vi "Test NI DAQ API.vi"() -> ()   [LabVIEW 2020]
doc: "NI DAQ API Tester."
uses:
  NI DAQ.lvlib
  <vilib>/Utility/error.llb/DialogType.ctl
  <resource>/objmgr/daqmx.rc
  Support/Task list.ctl
  Support/Continuous aquisition params.ctl
  <vilib>/Utility/miscctls.llb/LVRowAndColumnTypeDef.ctl
  AI config parameters--cluster.ctl
panel:
  in  "Task list":T1 caption="Task"
  in  "Channels available":i32(listbox)
  out "Waveform Chart":dbl[](graph)
  out "Digital data":bool[](array[boolean])
  out "Analog data":dbl[](array[numeric])
  in  "Stop continuous acquisition":bool
  in  "N samples":i32
  in  "Acquisition type":enum16{"Single", "Multiple"}(ring)=enum."Multiple"
  in  "Start continous acquisition":bool
  out "DevSerialNum":u32
  out "Connection valid?":bool
  in  "Validate connection":bool
  in  "Sleep HL":bool
  in  "Task list":T1=enum."DO task" caption="Task"
  in  "Timeout":i32=100
  in  "Wake up HL":bool
  in  "Task list 2":T1 caption="Task to get"
  out "DAQmx Task":refnum<k21>
  in  "Get task ref":bool
  in  "Tab Control":enum32{"DO", "DI", "AI", "AO", "CI"}(tab)
  in  "Write DO":bool
  in  "Samples":enum16{"Single", "Multiple"}(ring)
  in  "Data":bool[](array[boolean])
  in  "Create DO channel":bool
  in  "Create DI channel":bool
  in  "Samples 2":enum16{"Single", "Multiple"}(ring) caption="Samples"
  in  "Read DI":bool
  out "Data read":bool[](array[boolean])
  in  "Create AI channel":bool
  in  "Config params":T2={"Terminal configuration"=-1, "min value"=-5.0, "max value"=5.0} {"max value" format="%0.2f"; "min value" format="%0.2f"; "Terminal configuration" items=["Default"=-1, "RSE"=10083, "NRSE"=10078, "Differential"=10106, "Pseudodifferential"=12529]}
  in  "Read AI":bool
  in  "Samples 3":enum16{"Single", "Multiple"}(ring) caption="Samples"
  out "AI Data":dbl[](array[numeric])
  in  "Create AO channel":bool
  in  "Config params 2":T2={"Terminal configuration"=-1, "min value"=-5.0, "max value"=5.0} caption="Config params" {"max value" format="%0.2f"; "min value" format="%0.2f"; "Terminal configuration" items=["Default"=-1, "RSE"=10083, "NRSE"=10078, "Differential"=10106, "Pseudodifferential"=12529]}
  in  "Write AO":bool
  in  "Value(s)":dbl[](array[numeric])
  in  "Samples 4":enum16{"Single", "Multiple"}(ring) caption="Samples"
  in  "Create CI channel":bool
  in  "Channel config":T3={"Initial count"=0, "Count direction"=10128, "Edge"=10171} {"Count direction" items=["Count Up"=10128, "Count Down"=10124, "Externally Controlled"=10326]; "Edge" items=["Rising"=10280, "Falling"=10171]}
  in  "Read CI":bool
  in  "Samples 5":enum16{"Single", "Multiple"}(ring) caption="Samples"
  out "data":dbl[](array[numeric])
  in  "Stop task":bool
  in  "Start task":bool
  in  "Channel name":string
  in  "Physical channel(s)":string
  out "Available channels":i32(listbox)
  in  "Get channel list":bool
  in  "Set device ID":bool
  in  "Avilable devices":u16(ring) items=["Dev3", "Dev4", "Phys-6008"]
  in  "Show Diagram on Init":bool
  in  "Run as Singleton?":bool
  in  "Show Block Diagram":bool
  in  "Refresh Modules":bool
  out "Active Modules":string[](array[string])
  in  "Stop Module":bool
  in  "Select Module":i32(ring)=-1 caption="Select Module\nTo send Request to" items=["All"=-1]
  in  "Run New Module":bool
  in  "Hide Module Panel":bool
  in  "Show Module Panel":bool
  out "Status":string
  # "This VI tests the API for the Module."
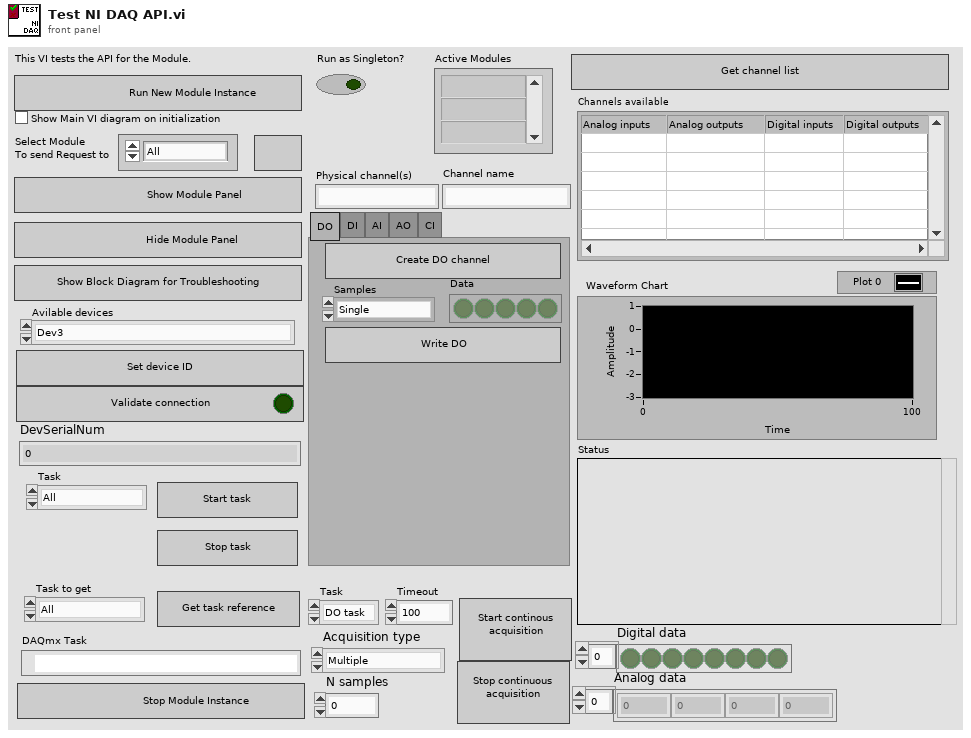
[diagram p1: front panel]
types:
  T1 = typedef "NI DAQ.lvlib/Task list.ctl" = enum16{"All", "DO task", "DI task", "AO task", "AI task", "CI task", "CO task"}
  T2 = typedef "NI DAQ.lvlib/AI config parameters--cluster.ctl" = cluster{"Terminal configuration":i32, "min value":dbl, "max value":dbl}
  T3 = cluster{"Initial count":u32, "Count direction":i32, "Edge":i32}
  T4 = typedef "LVRowAndColumnTypeDef.ctl" = cluster{"Row":i32, "Column":i32}
  T5 = typedef "NI DAQ.lvlib/Broadcast Events--cluster.ctl" = cluster{"Module Did Init":refnum<user-event>, "Status Updated":refnum<user-event>, "Error Reported":refnum<user-event>, "Module Did Stop":refnum<user-event>, "Update Module Execution Status":refnum<user-event>, "Digital data acquired":refnum<user-event>, "Device connected":refnum<user-event>, "Connection failed":refnum<user-event>, "Analog data acquired":refnum<user-event>, "Counter data acquired":refnum<user-event>}
  T6 = typedef "NI DAQ.lvlib/Continuous aquisition params.ctl" = cluster{"Module ID":i32, "Task list":T1, "Timeout":i32, "Acq type":enum16{"Single", "Multiple"}, "Data in":variant, "DAQmx Task":refnum<k21>, "N samples":i32}
  T7 = typedef "DialogType.ctl" = u16
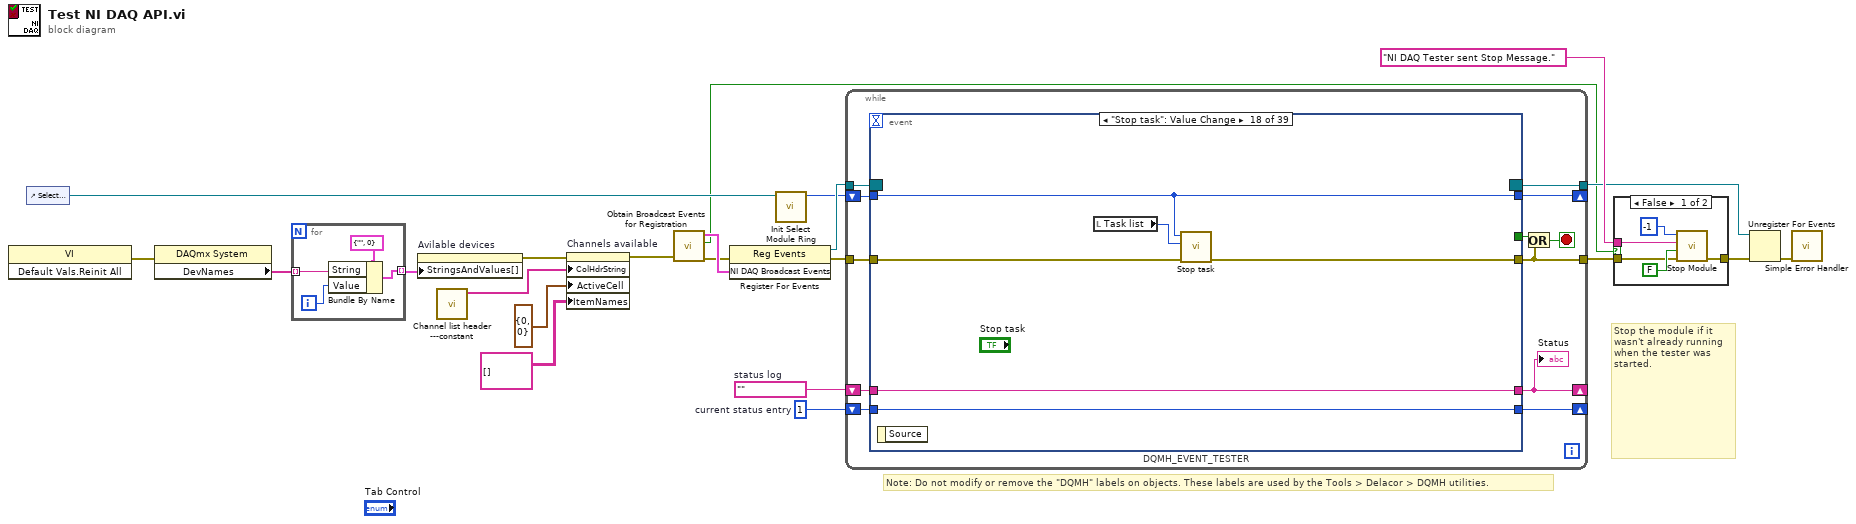
[diagram p0: block diagram]
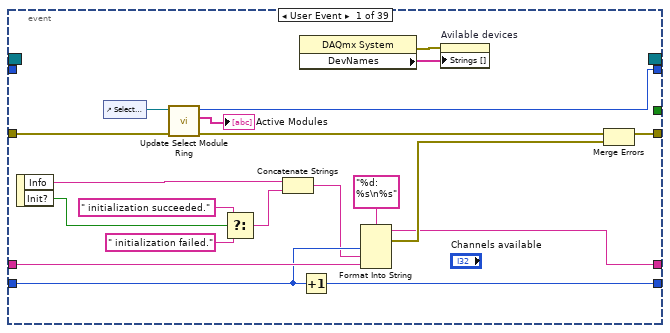
[diagram p3: hidden frame]
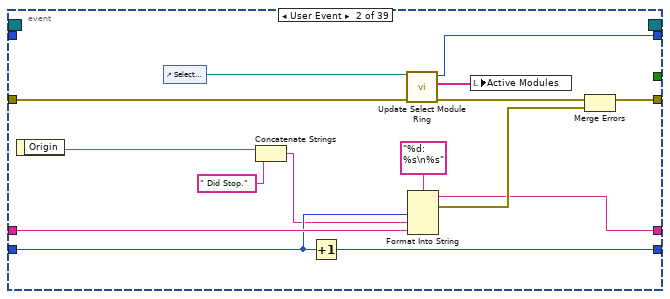
[diagram p4: hidden frame]
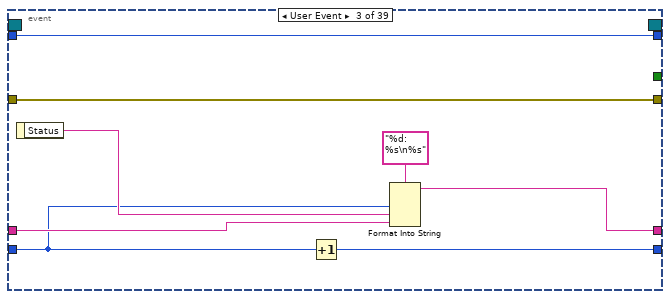
[diagram p5: hidden frame]
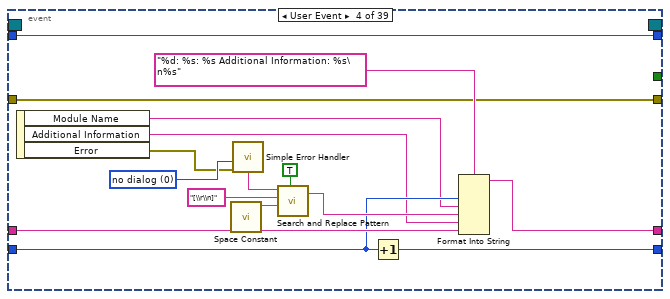
[diagram p6: hidden frame]
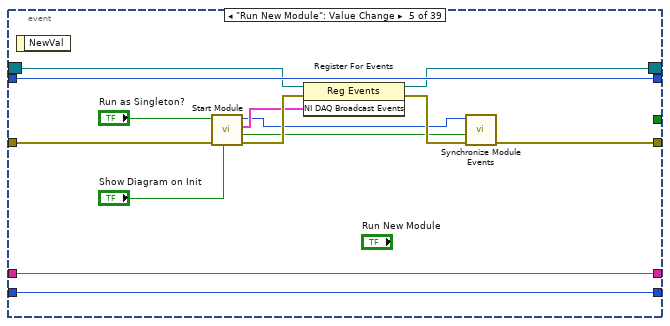
[diagram p7: hidden frame]
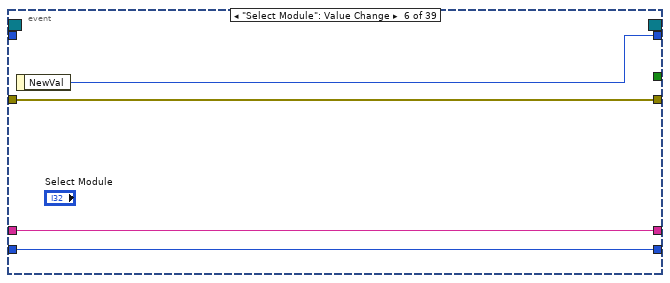
[diagram p8: hidden frame]
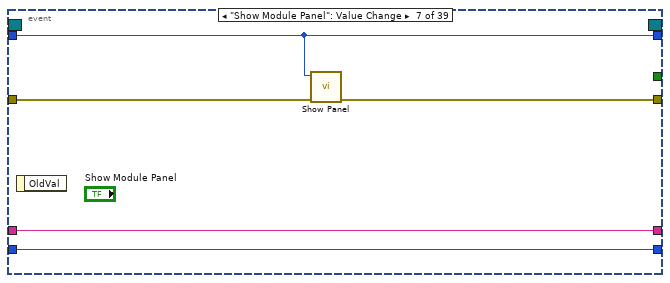
[diagram p9: hidden frame]
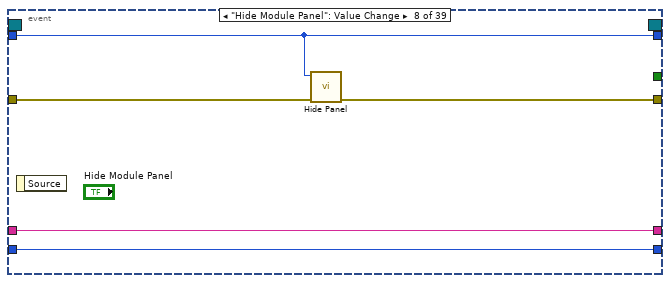
[diagram p10: hidden frame]
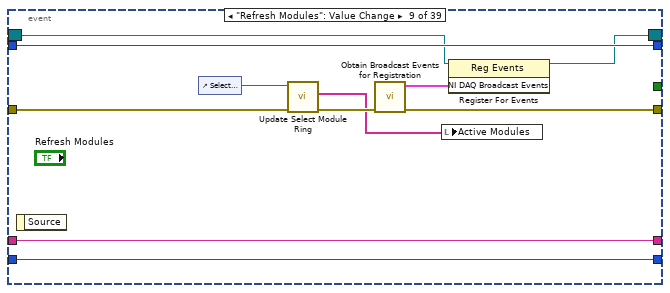
[diagram p11: hidden frame]
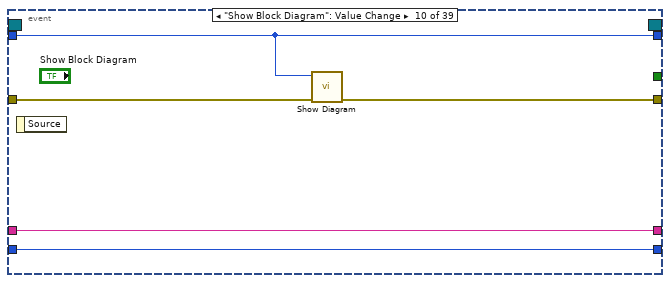
[diagram p12: hidden frame]
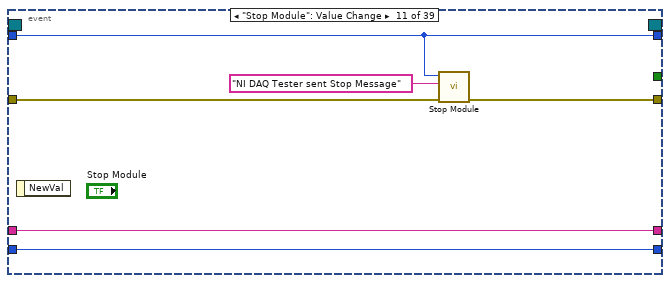
[diagram p13: hidden frame]
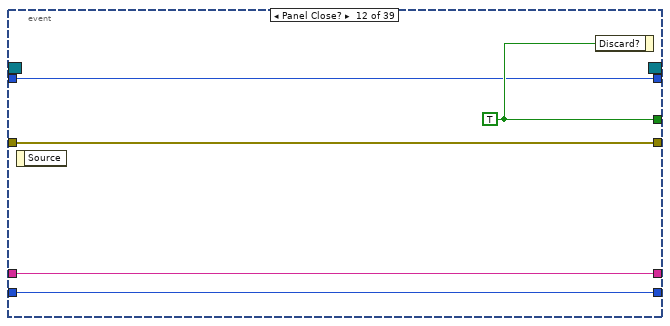
[diagram p14: hidden frame]
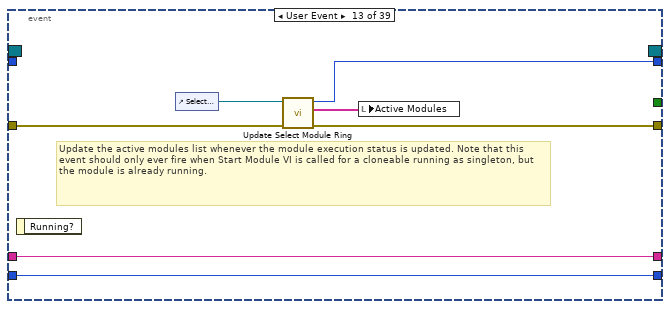
[diagram p15: hidden frame]
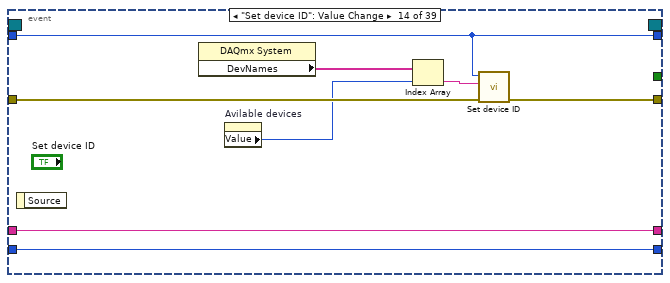
[diagram p16: hidden frame]
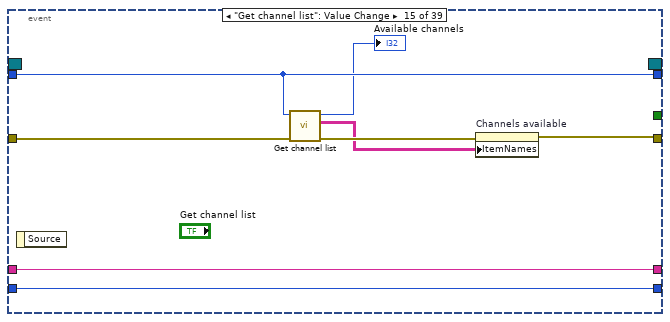
[diagram p17: hidden frame]
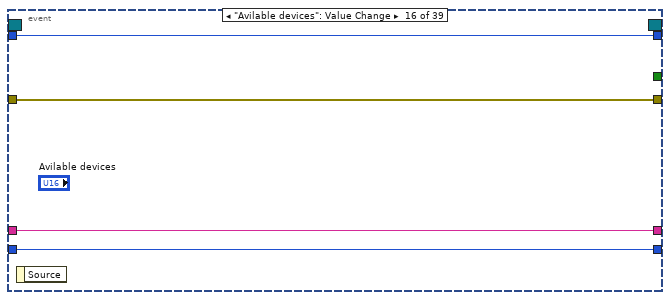
[diagram p18: hidden frame]
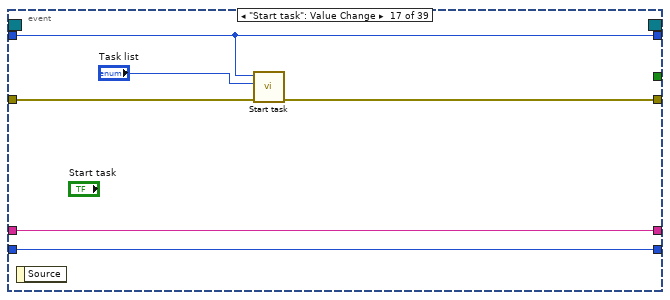
[diagram p19: hidden frame]
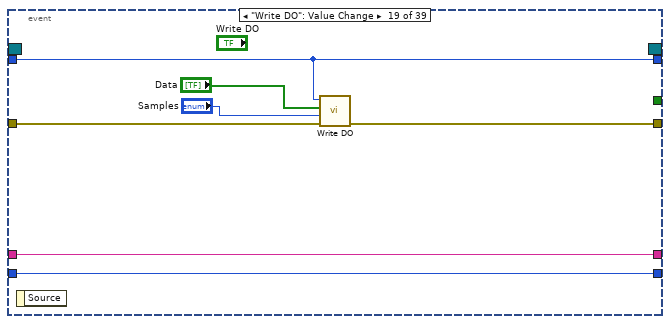
[diagram p20: hidden frame]
diagram:
  w19 = 1  # current status entry
  w20 = ""  # status log
  # "Stop the module if it wasn't already running when the tester was started."
  # "Note: Do not modify or remove the \"DQMH\" labels on objects. These labels are used by the Tools > Delacor > DQMH utilities."
  n1 = invoke class="VI" method="Default Vals.Reinit All"() -> (error out=w8:errorcluster)  [unwired: 3 in, 2 out]
  n2 = control-ref of="Select Module"() -> (w17:refnum<vi>)
  n3 = property class="DAQmx System"(error in=w8) -> ("DevNames"=w7:tag[])  [unwired: 1 in, 2 out]
  n4 = for {
    tunnel: w7 -> [w25] mode=indexing
    tunnel: [w23] -> w6 mode=indexing
    i -> [w24]
    n5 = Bundle By Name(cluster=cluster{"String":string, "Value":u16} {"String"="", "Value"=0} ("Cluster"), "String"=w25, "Value"=w24) -> (w23:cluster{"String":string, "Value":u16})
  }
  n6 = property on="Avilable devices" class="Ring (strict)"("StringsAndValues[]"=w6) -> (error out=w4:errorcluster)  [unwired: 2 in, 1 out]
  n7 = call "Channel list header ---constant.vi"() -> ("Column Header Strings"=w1:string[])  [unwired: 11 in]
  n8 = property on="Channels available" class="MCListbox (strict)"(error in=w4, "ColHdrString"=w1, "ActiveCell"=T4 {"Row"=0, "Column"=0} ("Active Cell:Active Cell"), "ItemNames"=string[][] [] ("Item Names")) -> (error out=w3:errorcluster)  [unwired: 1 in, 1 out]
  n9 = call "Obtain Broadcast Events for Registration.vi"("error in"=w3) -> ("error out"=w12:errorcluster, "Already running?"=w11:bool, "NI DAQ Broadcast Events"=w16:T5)  [unwired: 8 in]
  n10 = register-events(error in=w12, w16) -> (reference out=w22:refnum<event-registration>, error out=w15:errorcluster)  [unwired: 1 in]
  n11 = call "Init Select Module Ring.vi"("Select Module Ring Ref"=w17) -> ("Value for All Modules"=w18:i32)  [unwired: 8 in, 2 out]
  n12 = while {
    tunnel: w22 -> [w38]
    tunnel: [w27] -> w10
    tunnel: w15 -> [w36]
    shift-right: [w32] -> _
    shift-left: w20 -> [w34]
    shift-right: [w33] -> _
    shift-left: w19 -> [w35]
    shift-right: [w29] -> _
    shift-left: w18 -> [w30]
    tunnel: [w28] -> w13
    stop <- w31 stop-if-true
    n13 = event "DQMH_EVENT_TESTER" shown="[17] \"Stop task\": Value Change" {
      selector: w38 -> [_ _ _ _ w105 _ _ _ w131 _ _ _ _ _ _ _ _ _ _ _ _ _ _ _ _ _ _ _ _ _ _ _ _ _ _ _ _ _ _]
      dyn-events: [_ _ _ _ w104 _ _ _ w130 _ _ _ _ _ _ _ _ _ _ _ _ _ _ _ _ _ _ _ _ _ _ _ _ _ _ _ _ _ _] -> w28
      timeout: _ -> [_ _ _ _ _ _ _ _ _ _ _ _ _ _ _ _ _ _ _ _ _ _ _ _ _ _ _ _ _ _ _ _ _ _ _ _ _ _ _]
      tunnel: [_ _ _ _ _ _ _ _ _ _ _ w152 _ _ _ _ _ _ _ _ _ _ _ _ _ _ _ _ _ _ _ _ _ _ _ _ _ _ _] -> w37
      tunnel: [w49 w65 w81 w85 w103 w115 w119 w124 w127 w138 w143 w151 w155 w164 w169 w179 w182 w188 w195 w202 w209 w216 w230 w234 w248 w253 w260 w268 w275 w281 w295 w306 w312 w317 w331 w334 w342 w349 w363] -> w27
      tunnel: w36 -> [w50 w67 w81 w85 w106 w115 w120 w125 w132 w141 w144 w151 w156 w167 w175 w179 w185 w191 w198 w205 w212 w219 w229 w237 w248 w256 w263 w271 w278 w284 w295 w306 w315 w320 w331 w338 w346 w353 w363]
      tunnel: w35 -> [w55 w70 w74 w88 w108 w113 w117 w122 w135 w139 w146 w149 w158 w165 w173 w177 w183 w189 w196 w203 w210 w217 w231 w235 w244 w254 w261 w269 w276 w282 w291 w302 w313 w318 w327 w336 w344 w351 w359]
      tunnel: w34 -> [w56 w71 w77 w89 w109 w114 w118 w123 w136 w140 w147 w150 w159 w166 w174 w178 w184 w190 w197 w204 w211 w218 w232 w236 w246 w255 w262 w270 w277 w283 w293 w304 w314 w319 w329 w337 w345 w352 w361]
      tunnel: [w53 w68 w78 w87 w109 w114 w118 w123 w136 w140 w147 w150 w159 w166 w174 w178 w184 w190 w197 w204 w211 w218 w232 w236 w245 w255 w262 w270 w277 w283 w292 w303 w314 w319 w328 w337 w345 w352 w360] -> w32
      tunnel: [w54 w69 w80 w86 w108 w113 w117 w122 w135 w139 w146 w149 w158 w165 w173 w177 w183 w189 w196 w203 w210 w217 w231 w235 w243 w254 w261 w269 w276 w282 w290 w301 w313 w318 w326 w336 w344 w351 w358] -> w33
      tunnel: w30 -> [_ _ w75 w97 w107 _ w116 w121 w134 w137 w145 w148 _ w163 w172 w176 w181 w187 w194 w201 w208 w215 w227 w233 w247 w252 w259 w267 w274 w280 w294 w305 w311 w316 w330 w335 w343 w350 w362]
      tunnel: [w41 w62 w75 w97 w107 w112 w116 w121 w134 w137 w145 w148 w154 w163 w172 w176 w181 w187 w194 w201 w208 w215 w227 w233 w247 w252 w259 w267 w274 w280 w294 w305 w311 w316 w330 w335 w343 w350 w362] -> w29
      event User Event {
        n14 = event-data() -> ("Info"=w52:string, "Init?"=w44:bool)  [unwired: 1 in]
        n15 = control-ref of="Select Module"() -> (w48:refnum<vi>)
        n16 = call "Update Select Module Ring.vi"("error in (no error)"=w50, "Select Module Ring Ref"=w48) -> ("error out"=w42:errorcluster, "Active Modules (Array)"=→"Active Modules":string[], "New Module Ring Value"=w41:i32)  [unwired: 7 in]
        n17 = Select(t=" initialization succeeded.", s=w44, f=" initialization failed.") -> (s? t:f=w43:string)
        n18 = Concatenate Strings(w52, w43) -> (w51:string)
        n19 = property class="DAQmx System"() -> (error out=w40:errorcluster, "DevNames"=w39:tag[])  [unwired: 2 in, 1 out]
        n20 = Increment(x=w55) -> (x+1=w54:i32)
        n21 = Format Into String(format string="%d: %s\n%s", w55, w51, w56) -> (resulting string=w53:string, error out=w58:errorcluster)  [unwired: 2 in]
        n22 = property on="Avilable devices" class="Ring (strict)"(error in=w40, "Strings []"=w39) -> ()  [unwired: 1 in, 2 out]
        n23 = Merge Errors(w42, w58) -> (w49:errorcluster)
      }
      event User Event {
        n24 = event-data() -> ("Origin"=w60:string)  [unwired: 1 in]
        n25 = control-ref of="Select Module"() -> (w64:refnum<vi>)
        n26 = Concatenate Strings(w60, " Did Stop.") -> (w59:string)
        n27 = Increment(x=w70) -> (x+1=w69:i32)
        n28 = call "Update Select Module Ring.vi"("error in (no error)"=w67, "Select Module Ring Ref"=w64) -> ("error out"=w66:errorcluster, "Active Modules (Array)"=w63:string[], "New Module Ring Value"=w62:i32)  [unwired: 7 in]
        n29 = Format Into String(format string="%d: %s\n%s", w70, w59, w71) -> (resulting string=w68:string, error out=w73:errorcluster)  [unwired: 2 in]
        n30 = local write "Active Modules"(w63) -> ()
        n31 = Merge Errors(w66, w73) -> (w65:errorcluster)
      }
      event User Event {
        n32 = event-data() -> ("Status"=w76:string)  [unwired: 1 in]
        n33 = Increment(x=w74) -> (x+1=w80:i32)
        n34 = Format Into String(format string="%d: %s\n%s", w74, w76, w77) -> (resulting string=w78:string)  [unwired: 2 in, 1 out]
      }
      event User Event {
        w90 = T7 0 items=["no dialog", "OK message", "continue or stop message", "OK message + warnings", "continue/stop + warnings"] ("type of dialog (OK msg:1)")
        n35 = event-data() -> ("Module Name"=w84:string, "Additional Information"=w83:string, "Error"=w82:errorcluster)  [unwired: 1 in]
        n36 = call <vilib>:"Space Constant.vi"() -> ("String"=w94:string)
        n37 = call <vilib>:"Simple Error Handler.vi"("type of dialog (OK msg:1)"=w90, "error in (no error)"=w82) -> ("message"=w91:string)  [unwired: 3 in, 4 out]
        n38 = call <vilib>:"Search and Replace Pattern.vi"("string"=w91, "regular expression (\"\")"="[\\r\\n]" ("regular expression (\"\")"), "replace string (\"\")"=w94, "replace all? (F)"=TRUE ("replace all CR/LF with spaces")) -> ("result string"=w92:string)  [unwired: 1 in, 1 out]
        n39 = Increment(x=w88) -> (x+1=w86:i32)
        n40 = Format Into String(format string="%d: %s: %s Additional Information: %s\n%s", w88, w84, w92, w83, w89) -> (resulting string=w87:string)  [unwired: 2 in, 1 out]
      }
      event "Run New Module": Value Change {
        n41 = event-data() -> ()  [unwired: 1 in, 1 out]
        n42 = call "Start Module.vi"("Show Main VI Diagram on Init (F)"="Show Diagram on Init", "error in"=w106, "Run as Singleton? (F)"="Run as Singleton?") -> ("error out"=w110:errorcluster, "Wait for Event Sync?"=w102:bool, "NI DAQ Broadcast Events"=w101:T5, "Module ID"=w98:i32)  [unwired: 5 in]
        n43 = register-events(reference=w105, error in=w110, w101) -> (reference out=w104:refnum<event-registration>, error out=w111:errorcluster)
        n44 = call "Synchronize Module Events.vi"("error in"=w111, "Wait for Event Sync?"=w102, "Module ID in"=w98) -> ("error out"=w103:errorcluster)  [unwired: 7 in, 1 out]
      }
      event "Select Module": Value Change {
        n45 = event-data() -> ("NewVal"=w112:i32)  [unwired: 1 in]
      }
      event "Show Module Panel": Value Change {
        n46 = event-data() -> ()  [unwired: 1 in, 1 out]
        n47 = call "Show Panel.vi"("error in (no error)"=w120, "Module ID"=w116) -> ("error out"=w119:errorcluster)  [unwired: 9 in]
      }
      event "Hide Module Panel": Value Change {
        n48 = event-data() -> ()  [unwired: 1 in, 1 out]
        n49 = call "Hide Panel.vi"("error in (no error)"=w125, "Module ID"=w121) -> ("error out"=w124:errorcluster)  [unwired: 9 in]
      }
      event "Refresh Modules": Value Change {
        n50 = event-data() -> ()  [unwired: 1 in, 1 out]
        n51 = control-ref of="Select Module"() -> (w133:refnum<vi>)
        n52 = call "Update Select Module Ring.vi"("error in (no error)"=w132, "Select Module Ring Ref"=w133) -> ("error out"=w128:errorcluster, "Active Modules (Array)"=w126:string[])  [unwired: 7 in, 1 out]
        n53 = call "Obtain Broadcast Events for Registration.vi"("error in"=w128) -> ("error out"=w127:errorcluster, "NI DAQ Broadcast Events"=w129:T5)  [unwired: 8 in, 1 out]
        n54 = local write "Active Modules"(w126) -> ()
        n55 = register-events(reference=w131, w129) -> (reference out=w130:refnum<event-registration>)  [unwired: 1 in, 1 out]
      }
      event "Show Block Diagram": Value Change {
        n56 = event-data() -> ()  [unwired: 1 in, 1 out]
        n57 = call "Show Diagram.vi"("error in (no error)"=w141, "Module ID"=w137) -> ("error out"=w138:errorcluster)  [unwired: 9 in]
      }
      event "Stop Module": Value Change {
        n58 = event-data() -> ()  [unwired: 1 in, 1 out]
        n59 = call "Stop Module.vi"("error in"=w144, "Origin"="NI DAQ Tester sent Stop Message", "Module ID"=w145) -> ("error out"=w143:errorcluster)  [unwired: 8 in]
      }
      event Panel Close? {
        w152 = TRUE ("Discard?")
        n60 = event-data() -> ()  [unwired: 1 in, 1 out]
        n61 = event-data("Discard?"=w152) -> ()  [unwired: 1 in, 1 out]
      }
      event User Event {
        # "Update the active modules list whenever the module execution status is updated. Note that this event should only ever fire when Start Module VI is called for a cloneable running as singleton, but the module is already running."
        n62 = event-data() -> ()  [unwired: 1 in, 1 out]
        n63 = control-ref of="Select Module"() -> (w157:refnum<vi>)
        n64 = call "Update Select Module Ring.vi"("error in (no error)"=w156, "Select Module Ring Ref"=w157) -> ("error out"=w155:errorcluster, "Active Modules (Array)"=w153:string[], "New Module Ring Value"=w154:i32)  [unwired: 7 in]
        n65 = local write "Active Modules"(w153) -> ()
      }
      event "Set device ID": Value Change {
        n66 = event-data() -> ()  [unwired: 1 in, 1 out]
        n67 = property class="DAQmx System"() -> ("DevNames"=w160:tag[])  [unwired: 2 in, 2 out]
        n68 = property on="Avilable devices" class="Ring (strict)"() -> ("Value"=w162:u16)  [unwired: 2 in, 2 out]
        n69 = Index Array(array=w160, index=w162) -> (element=w161:tag)
        n70 = call "Set device ID.vi"("error in"=w167, "Device ID"=w161, "Module ID"=w163) -> ("error out"=w164:errorcluster)  [unwired: 8 in]
      }
      event "Get channel list": Value Change {
        n71 = event-data() -> ()  [unwired: 1 in, 1 out]
        n72 = call "Get channel list.vi"("error in"=w175, "Module ID"=w172) -> ("error out"=w170:errorcluster, "Available channels 2"=w168:string[][], "Available channels"=→"Available channels":i32)  [unwired: 6 in, 1 out]
        n73 = property on="Channels available" class="MCListbox (strict)"(error in=w170, "ItemNames"=w168) -> (error out=w169:errorcluster)  [unwired: 1 in, 1 out]
      }
      event "Avilable devices": Value Change {
        n74 = event-data() -> ()  [unwired: 1 in, 1 out]
      }
      event "Start task": Value Change {
        n75 = event-data() -> ()  [unwired: 1 in, 1 out]
        n76 = call "Start task.vi"("error in"=w185, "Task list"="Task list", "Module ID"=w181) -> ("error out"=w182:errorcluster)  [unwired: 8 in]
      }
      event "Stop task": Value Change {
        n77 = event-data() -> ()  [unwired: 1 in, 1 out]
        n78 = local read "Task list"() -> (w186:T1)
        n79 = call "Stop task.vi"("error in"=w191, "Task list"=w186, "Module ID"=w187) -> ("error out"=w188:errorcluster)  [unwired: 8 in]
      }
      event "Write DO": Value Change {
        n80 = event-data() -> ()  [unwired: 1 in, 1 out]
        n81 = call "Write DO.vi"("error in"=w198, "Samples"="Samples", "Data"="Data", "Module ID"=w194) -> ("error out"=w195:errorcluster)  [unwired: 7 in]
      }
      event "Create DI channel": Value Change {
        n82 = event-data() -> ()  [unwired: 1 in, 1 out]
        n83 = local read "Channel name"() -> (w199:string)
        n84 = local read "Physical channel(s)"() -> (w200:string)
        n85 = call "Create DI channel.vi"("error in"=w205, "Channel name"=w199, "Physical channel"=w200, "Module ID"=w201) -> ("error out"=w202:errorcluster)  [unwired: 7 in]
      }
      event "Read DI": Value Change {
        n86 = event-data() -> ()  [unwired: 1 in, 1 out]
        n87 = call "Read DI.vi"("error in"=w212, "Samples"="Samples 2", "Module ID"=w208) -> ("error out"=w209:errorcluster, "Data"=→"Data read":bool[])  [unwired: 6 in, 1 out]
      }
      event "Get task ref": Value Change {
        n88 = event-data() -> ()  [unwired: 1 in, 1 out]
        n89 = call "Get task ref.vi"("error in"=w219, "Task list"="Task list 2", "Module ID"=w215) -> ("error out"=w216:errorcluster, "DAQmx Task"=→"DAQmx Task":refnum<k21>)  [unwired: 6 in, 1 out]
      }
      event "Wake up HL": Value Change {
        n90 = event-data() -> ()  [unwired: 1 in, 1 out]
        n91 = call "Get task ref.vi"("error in"=w229, "Task list"="Task list", "Module ID"=w227) -> ("error out"=w228:errorcluster)  [unwired: 6 in, 2 out]
        n92 = local read "Data"() -> (w224:bool[])
        n93 = Bundle By Name(cluster=T6 {"Module ID"=0, "Task list"=enum."All", "Timeout"=0, "Acq type"=enum."Single", "Data in"=variant, "DAQmx Task"="", "N samples"=0} ("Acquisition data"), "Task list"="Task list", "Timeout"="Timeout", "Acq type"=enum16{"Single", "Multiple"}."Multiple" ("Samples"), "Data in"=w224) -> (w220:T6)
        n94 = call "Wake up HL.vi"("wait for reply (T)"=FALSE, "error in"=w228, "Acquisition data"=w220, "Module ID"=w227) -> ("error out"=w230:errorcluster)  [unwired: 5 in, 2 out]
      }
      event "Sleep HL": Value Change {
        n95 = event-data() -> ()  [unwired: 1 in, 1 out]
        n96 = call "Sleep HL.vi"("error in"=w237, "Module ID"=w233) -> ("error out"=w234:errorcluster)  [unwired: 9 in]
      }
      event User Event {
        n97 = event-data() -> ("Data"=→"Digital data":bool[])  [unwired: 1 in]
        n98 = Format Into String(format string="Response Received - %s", "Data acquired." ("input 1")) -> (resulting string=w240:string)  [unwired: 2 in, 1 out]
        n99 = Increment(x=w244) -> (x+1=w243:i32)
        n100 = Format Into String(format string="%d: %s\n%s", w244, w240, w246) -> (resulting string=w245:string)  [unwired: 2 in, 1 out]
      }
      event "Create AI channel": Value Change {
        n101 = event-data() -> ()  [unwired: 1 in, 1 out]
        n102 = local read "Channel name"() -> (w250:string)
        n103 = local read "Physical channel(s)"() -> (w251:string)
        n104 = call "Create AI channel.vi"("Config params"="Config params", "error in"=w256, "Channel name"=w250, "Physical channel"=w251, "Module ID"=w252) -> ("error out"=w253:errorcluster)  [unwired: 6 in]
      }
      event "Read AI": Value Change {
        n105 = event-data() -> ()  [unwired: 1 in, 1 out]
        n106 = call "Read AI.vi"("error in"=w263, "Samples"="Samples 3", "Module ID"=w259) -> ("error out"=w260:errorcluster, "Data"=→"AI Data":dbl[])  [unwired: 6 in, 1 out]
      }
      event "Create AO channel": Value Change {
        n107 = event-data() -> ()  [unwired: 1 in, 1 out]
        n108 = local read "Channel name"() -> (w265:string)
        n109 = local read "Physical channel(s)"() -> (w266:string)
        n110 = call "Create AO channel.vi"("Config params"="Config params 2", "error in"=w271, "Channel name"=w265, "Physical channel"=w266, "Module ID"=w267) -> ("error out"=w268:errorcluster)  [unwired: 6 in]
      }
      event "Write AO": Value Change {
        n111 = event-data() -> ()  [unwired: 1 in, 1 out]
        n112 = call "Write AO.vi"("error in"=w278, "Samples"="Samples 4", "Value(s)"="Value(s)", "Module ID"=w274) -> ("error out"=w275:errorcluster)  [unwired: 7 in]
      }
      event "Validate connection": Value Change {
        n113 = event-data() -> ()  [unwired: 1 in, 1 out]
        n114 = call "Validate connection.vi"("error in"=w284, "Module ID"=w280) -> ("error out"=w281:errorcluster, "DevSerialNum"=→"DevSerialNum":u32)  [unwired: 7 in, 1 out]
      }
      event User Event {
        n115 = event-data() -> ("Connected?"=→"Connection valid?":bool)  [unwired: 1 in]
        n116 = Format Into String(format string="Response Received - %s", "Device connected" ("input 1")) -> (resulting string=w287:string)  [unwired: 2 in, 1 out]
        n117 = Increment(x=w291) -> (x+1=w290:i32)
        n118 = Format Into String(format string="%d: %s\n%s", w291, w287, w293) -> (resulting string=w292:string)  [unwired: 2 in, 1 out]
      }
      event User Event {
        n119 = event-data() -> ("Connected?"=w297:bool)  [unwired: 1 in]
        n120 = local write "Connection valid?"(w297) -> ()
        n121 = Format Into String(format string="Response Received - %s", "Connection failed." ("input 1")) -> (resulting string=w298:string)  [unwired: 2 in, 1 out]
        n122 = Increment(x=w302) -> (x+1=w301:i32)
        n123 = Format Into String(format string="%d: %s\n%s", w302, w298, w304) -> (resulting string=w303:string)  [unwired: 2 in, 1 out]
      }
      event "Start continous acquisition": Value Change {
        n124 = event-data() -> ()  [unwired: 1 in, 1 out]
        n125 = local read "Task list"() -> (w309:T1)
        n126 = local read "Timeout"() -> (w308:i32)
        n127 = call "Start continous acquisition.vi"("N samples"="N samples", "Samples"="Acquisition type", "error in"=w315, "Timeout"=w308, "Task list"=w309, "Module ID"=w311) -> ("error out"=w312:errorcluster)  [unwired: 5 in]
      }
      event "Stop continuous acquisition": Value Change {
        n128 = event-data() -> ()  [unwired: 1 in, 1 out]
        n129 = call "Stop continuous acquisition.vi"("error in"=w320, "Module ID"=w316) -> ("error out"=w317:errorcluster)  [unwired: 9 in]
      }
      event User Event {
        n130 = event-data() -> ("Data"=→"Analog data" →"Waveform Chart":dbl[])  [unwired: 1 in]
        n131 = Format Into String(format string="Response Received - %s", "Analog data acquired." ("input 1")) -> (resulting string=w323:string)  [unwired: 2 in, 1 out]
        n132 = Increment(x=w327) -> (x+1=w326:i32)
        n133 = Format Into String(format string="%d: %s\n%s", w327, w323, w329) -> (resulting string=w328:string)  [unwired: 2 in, 1 out]
      }
      event "Create DO channel": Value Change {
        n134 = event-data() -> ()  [unwired: 1 in, 1 out]
        n135 = call "Create DO channel.vi"("error in"=w338, "Channel name"="Channel name", "lines"="Physical channel(s)", "Module ID"=w335) -> ("error out"=w334:errorcluster)  [unwired: 7 in]
      }
      event "Create CI channel": Value Change {
        n136 = event-data() -> ()  [unwired: 1 in, 1 out]
        n137 = local read "Physical channel(s)"() -> (w341:string)
        n138 = local read "Channel name"() -> (w340:string)
        n139 = call "Create CI channel.vi"("Channel config"="Channel config", "error in"=w346, "Channel name"=w340, "Physical channel"=w341, "Module ID"=w343) -> ("error out"=w342:errorcluster)  [unwired: 6 in]
      }
      event "Read CI": Value Change {
        n140 = event-data() -> ()  [unwired: 1 in, 1 out]
        n141 = call "Read CI.vi"("error in"=w353, "Samples"="Samples 5", "Module ID"=w350) -> ("error out"=w349:errorcluster, "data"=→"data":dbl[])  [unwired: 6 in, 1 out]
      }
      event User Event {
        # "#DQMH_CodeNeeded\n1. Process the event data sent by the \"Counter data acquired\" broadcast event.\n2. Delete or edit this label when done."
        n142 = event-data() -> ()  [unwired: 1 in, 6 out]
        n143 = Format Into String(format string="Response Received - %s", "Counter information available." ("input 1")) -> (resulting string=w355:string)  [unwired: 2 in, 1 out]
        n144 = Increment(x=w359) -> (x+1=w358:i32)
        n145 = Format Into String(format string="%d: %s\n%s", w359, w355, w361) -> (resulting string=w360:string)  [unwired: 2 in, 1 out]
      }
    }
    "Status" <- w32
    n146 = Or(x=w37, y=w27) -> (x .or. y?=w31:bool)
  }
  n147 = case shown="False" w11 {
    tunnel: [w368 w369] -> w21
    tunnel: "NI DAQ Tester sent Stop Message." ("Origin") -> [w367 _]
    tunnel: w10 -> [w364 w369]
    frame False {
      n148 = call "Stop Module.vi"("error in"=w364, "Wait for Module to stop? (F)"=FALSE ("Wait for Module to stop?"), "Origin"=w367, "Module ID"=-1 ("Stop all")) -> ("error out"=w368:errorcluster)  [unwired: 7 in]
    }
    frame True {
    }
  }
  n149 = Unregister For Events(event registration refnum=w13, error in=w21) -> (error out=w9:errorcluster)
  n150 = call <vilib>:"Simple Error Handler.vi"("error in (no error)"=w9) -> ()  [unwired: 4 in, 5 out]
